vi "Done.vi"(8 "error in (no error)":errorcluster, 11 "Text File Sink in":refnum<class "Text File Sink.lvclass">) -> (0 "error out":errorcluster, 3 "Text File Sink out":refnum<class "Text File Sink.lvclass">)   [LabVIEW 2016, in "Stream Log.lvlib" / "Text File Sink.lvclass"]
doc: "--\nCopyright © 2017 Composed SystemsI All rights reserved.\n\nAuthor: Jon McBee <jon.mcbee@composed.io>\n\nThis library is provided \"AS IS\" ,WITHOUT WARRANTIES OR\nCONDITIONS OF ANY KIND, either express or implied.\n\nComposed Systems -- composed.io\n\nStream 0.0.1.1\nJon McBee - Composed Systems\nCopyright (c) 2017, Composed Systems"
uses:
  <userlib>/Composed Systems/Stream/Log/Text File Sink/Text File Sink.lvclass
  <userlib>/Composed Systems/Stream/Log/Text File Sink/Text File Sink.lvclass/Text File Sink.ctl
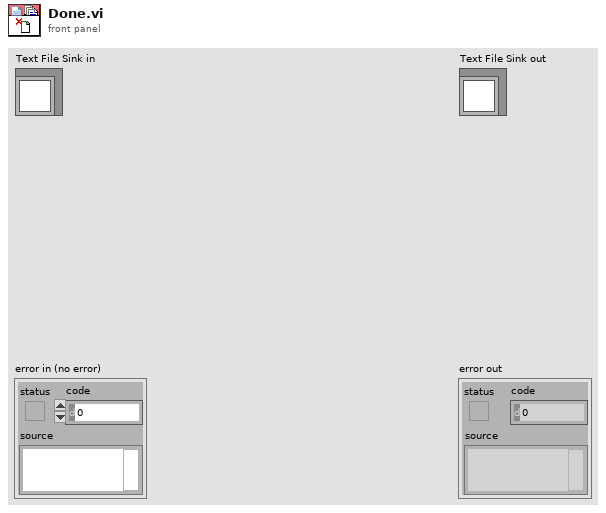
[diagram p1: front panel]
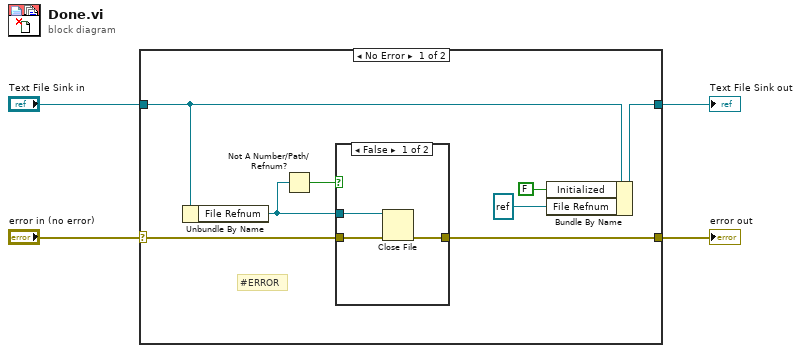
[diagram p0: block diagram]
diagram:
  n1 = case shown="No Error" "error in (no error)" {
    selector: "error in (no error)" -> [w9 w17]
    tunnel: [w8 w17] -> w3
    tunnel: [w6 w18] -> w2
    tunnel: "Text File Sink in" -> [w7 w18]
    frame No Error {
      # "#ERROR"
      n2 = Unbundle By Name(w7) -> ("File Refnum"=w11:refnum<file>)
      n3 = Not A Number/Path/Refnum?(number/path/refnum=w11) -> (NaN/Path/Refnum?=w10:bool)
      n4 = case shown="False" w10 {
        tunnel: w9 -> [w15 w16]
        tunnel: [w14 w16] -> w8
        tunnel: w11 -> [w13 _]
        frame False {
          n5 = Close File(refnum=w13, error in=w15) -> (error out=w14:errorcluster)  [unwired: 1 out]
        }
        frame True {
        }
      }
      n6 = Bundle By Name(cluster=w7, "Initialized"=FALSE, "File Refnum"=refnum<file> refnum) -> (w6:refnum<class "Text File Sink.lvclass">)
    }
    frame Error {
    }
  }
  "error out" <- w3
  "Text File Sink out" <- w2
